vi "Add Word Device.vi"(8 "error in (no error)":errorcluster, 9 "Device <JSON>":string, 10 "Device Code":string, 11 "SLMP in":refnum<class "SLMP.lvclass">) -> (0 "error out":errorcluster, 3 "SLMP out":refnum<class "SLMP.lvclass">)   [LabVIEW 2019, in "SLMP.lvlib" / "SLMP.lvclass"]
uses:
  SLMP.lvclass
  <vilib>/JDP Science/JSONtext/JSONtext.lvlib
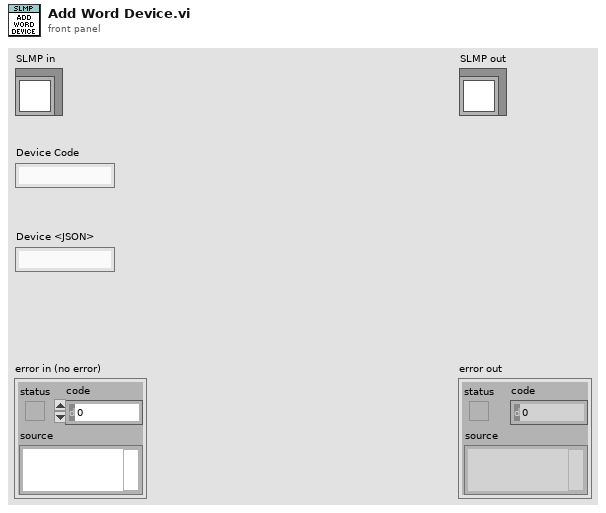
[diagram p1: front panel]
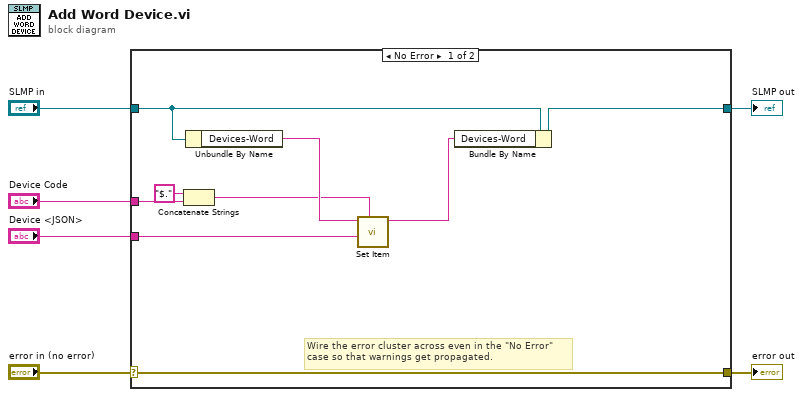
[diagram p0: block diagram]
diagram:
  n1 = case shown="No Error" "error in (no error)" {
    selector: "error in (no error)" -> [w15 w17]
    tunnel: [w15 w17] -> w5
    tunnel: [w8 w16] -> w3
    tunnel: "SLMP in" -> [w14 w16]
    tunnel: "Device Code" -> [w12 _]
    tunnel: "Device <JSON>" -> [w9 _]
    frame No Error {
      # "Wire the error cluster across even in the \"No Error\"\ncase so that warnings get propagated."
      n2 = Concatenate Strings("$." ("string"), w12) -> (w10:string)
      n3 = Unbundle By Name(w14) -> ("Devices-Word"=w13:string)
      n4 = call <vilib>:"Set Item.vi"("$Path or Item Name"=w10, "JSON to Insert"=w9, "JSON"=w13) -> ("<JSON>"=w7:string)  [unwired: 5 in, 2 out]
      n5 = Bundle By Name(cluster=w14, "Devices-Word"=w7) -> (w8:refnum<class "SLMP.lvclass">)
    }
    frame Error {
    }
  }
  "error out" <- w5
  "SLMP out" <- w3
